vi "cal_trans.vi"(0 "Reference":T1, 3 "Input":T2) -> ()   [LabVIEW 2024]
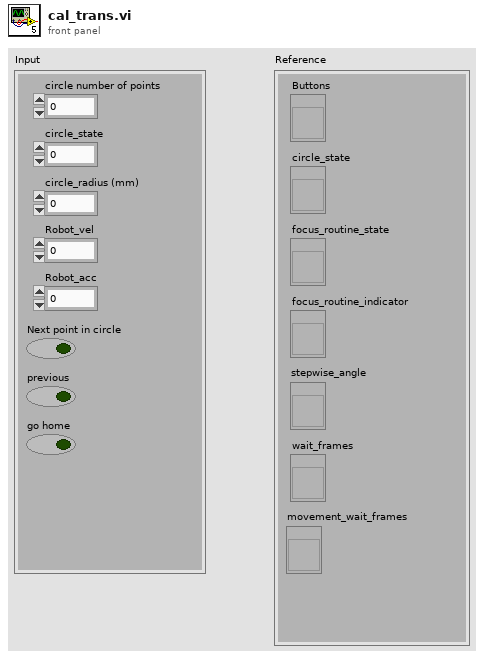
[diagram p1: front panel]
types:
  T1 = cluster{"Buttons":refnum<vi>, "circle_state":refnum<vi>, "focus_routine_state":refnum<vi>, "focus_routine_indicator":refnum<vi>, "stepwise_angle":refnum<vi>, "wait_frames":refnum<vi>, "movement_wait_frames":refnum<vi>}
  T2 = cluster{"circle number of points":i8, "circle_state":i8, "circle_radius (mm)":dbl, "Robot_vel":dbl, "Robot_acc":dbl, "Next point in circle":bool, "previous":bool, "go home":bool}
  T3 = cluster{"Focus routine":bool, "Freedrive mode":bool, "Next point in circle":bool, "previous":bool, "go home":bool}
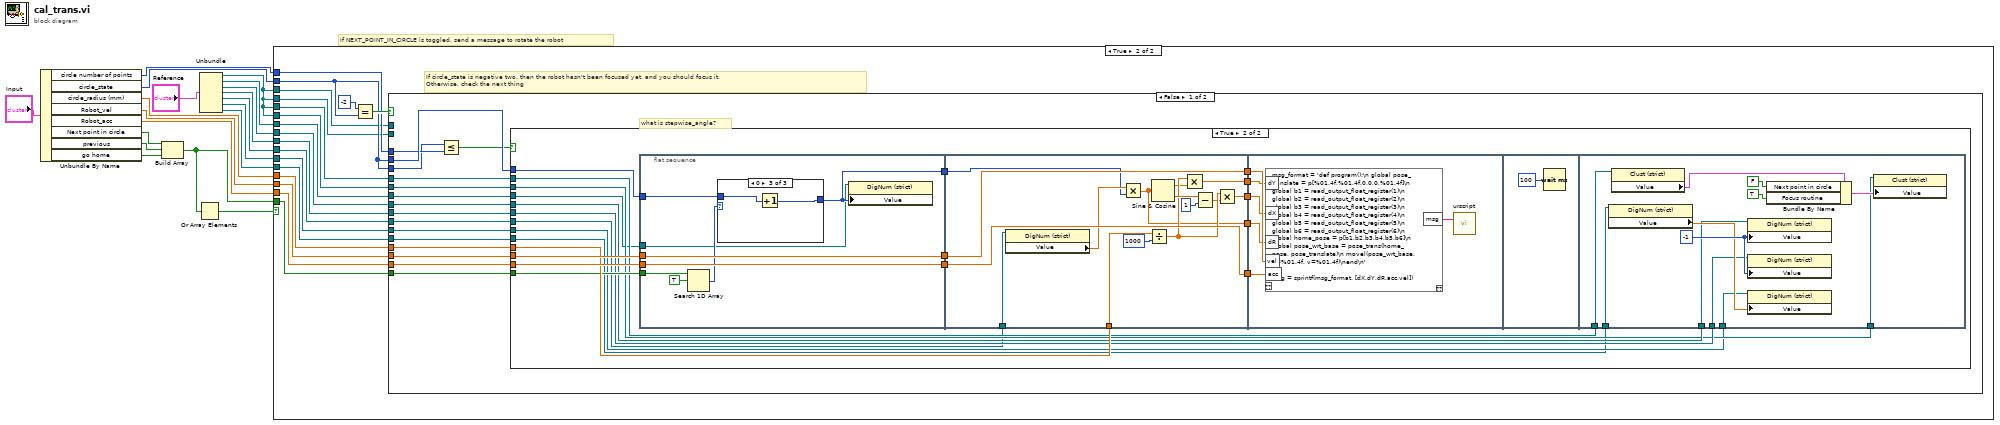
[diagram p0: block diagram]
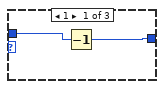
[diagram p4: hidden frame]
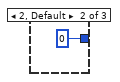
[diagram p5: hidden frame]
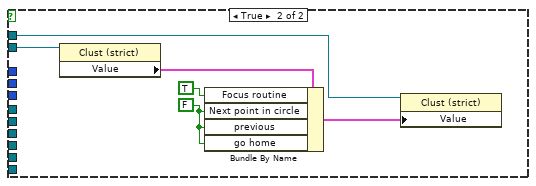
[diagram p6: hidden frame]
diagram:
  # "If NEXT_POINT_IN_CIRCLE is toggled, send a message to rotate the robot"
  n1 = Unbundle By Name("Input") -> ("circle number of points"=w16:i8, "circle_state"=w15:i8, "circle_radius (mm)"=w14:dbl, "Robot_vel"=w13:dbl, "Robot_acc"=w12:dbl, "Next point in circle"=w11:bool, "previous"=w9:bool, "go home"=w10:bool)
  n2 = Build Array(w11, w9, w10) -> (w19:bool[])
  n3 = Or Array Elements(Boolean array=w19) -> (logical OR=w18:bool)
  n4 = Unbundle("Reference") -> ("Buttons"=w7:refnum<vi>, "circle_state"=w6:refnum<vi>, "focus_routine_state"=w5:refnum<vi>, "focus_routine_indicator"=w4:refnum<vi>, "stepwise_angle"=w3:refnum<vi>, "wait_frames"=w2:refnum<vi>, "movement_wait_frames"=w1:refnum<vi>)
  n5 = case shown="True" w18 {
    tunnel: w15 -> [_ w32]
    tunnel: w16 -> [_ w35]
    tunnel: w13 -> [_ w34]
    tunnel: w12 -> [_ w33]
    tunnel: w14 -> [_ w31]
    tunnel: w19 -> [_ w30]
    tunnel: w5 -> [_ w29]
    tunnel: w4 -> [_ w28]
    tunnel: w7 -> [_ w27]
    tunnel: w2 -> [_ w26]
    tunnel: w1 -> [_ w25]
    tunnel: w7 -> [_ w24]
    tunnel: w3 -> [_ w23]
    tunnel: w6 -> [_ w22]
    tunnel: w7 -> [_ w21]
    tunnel: w7 -> [_ w20]
    frame False {
    }
    frame True {
      # "If circle_state is negative two, then the robot hasn't been focused yet, and you should focus it.\nOtherwise, check the next thing"
      n6 = Equal?(x=-2, y=w32) -> (x = y?=w36:bool)
      n7 = case shown="False" w36 {
        tunnel: w35 -> [w49 _]
        tunnel: w32 -> [w48 _]
        tunnel: w34 -> [w53 _]
        tunnel: w33 -> [w52 _]
        tunnel: w32 -> [w51 _]
        tunnel: w31 -> [w50 _]
        tunnel: w30 -> [w46 _]
        tunnel: w29 -> [w45 _]
        tunnel: w28 -> [w44 _]
        tunnel: w27 -> [w43 _]
        tunnel: w26 -> [w42 _]
        tunnel: w25 -> [w41 _]
        tunnel: w24 -> [w40 _]
        tunnel: w23 -> [w39 _]
        tunnel: w22 -> [w38 _]
        tunnel: w21 -> [_ w123]
        tunnel: w20 -> [_ w122]
        frame False {
          # "what is stepwise_angle?"
          n8 = Less Or Equal?(x=w48, y=w49) -> (x <= y?=w47:bool)
          n9 = case shown="True" w47 {
            tunnel: w53 -> [_ w74]
            tunnel: w52 -> [_ w73]
            tunnel: w51 -> [_ w64]
            tunnel: w50 -> [_ w65]
            tunnel: w46 -> [_ w62]
            tunnel: w45 -> [_ w61]
            tunnel: w44 -> [_ w60]
            tunnel: w43 -> [_ w59]
            tunnel: w42 -> [_ w58]
            tunnel: w41 -> [_ w57]
            tunnel: w40 -> [_ w56]
            tunnel: w39 -> [_ w55]
            tunnel: w38 -> [_ w54]
            frame False {
            }
            frame True {
              n10 = flat-sequence {
                tunnel: w64 -> [w80]
                tunnel: w73 -> [w81]
                tunnel: w74 -> [w82]
                tunnel: [w82] -> w67
                tunnel: [w81] -> w66
                tunnel: [w76] -> w63
                tunnel: w62 -> [w79]
                tunnel: w54 -> [w75]
                tunnel: [w102] -> w72
                tunnel: [w101] -> w71
                tunnel: [w90] -> w70
                tunnel: [w91] -> w69
                tunnel: [w92] -> w68
                tunnel: w67 -> [w102]
                tunnel: w66 -> [w101]
                tunnel: w65 -> [w94]
                tunnel: w63 -> [w89]
                tunnel: w55 -> [w88]
                tunnel: w72 -> [w108]
                tunnel: w71 -> [w107]
                tunnel: w70 -> [w106]
                tunnel: w69 -> [w105]
                tunnel: w68 -> [w104]
                tunnel: w61 -> [w115]
                tunnel: w60 -> [w114]
                tunnel: w59 -> [w113]
                tunnel: w58 -> [w112]
                tunnel: w57 -> [w111]
                tunnel: w56 -> [w110]
                frame #0 {
                  n11 = Search 1D Array(1D array=w79, element=TRUE) -> (index of element=w77:i32)  [unwired: 1 in]
                  n12 = case shown="0" w77 {
                    tunnel: w80 -> [w84 _ w87]
                    tunnel: [w83 0 w86] -> w76
                    frame 1 {
                      n13 = Decrement(x=w84) -> (x-1=w83:i8)
                    }
                    frame 2, Default {
                    }
                    frame 0 {
                      n14 = Increment(x=w87) -> (x+1=w86:i8)
                    }
                  }
                  n15 = property class="DigNum (strict)"(reference=w75, "Value"=w76) -> ()  [unwired: 1 in, 2 out]
                }
                frame #1 {
                  n16 = property class="DigNum (strict)"(reference=w88) -> ("Value"=w96:dbl)  [unwired: 1 in, 2 out]
                  n17 = Multiply(x=w96, y=w89) -> (x*y=w90:dbl)
                  n18 = Divide(x=w94, y=1000) -> (x/y=w99:dbl)
                  n19 = Sine & Cosine(0:w90) -> (1:w97:dbl, 2:w100:dbl)
                  n20 = Multiply(x=w99, y=w97) -> (x*y=w91:dbl)
                  n21 = Subtract(x=w100, y=1) -> (x-y=w98:dbl)
                  n22 = Multiply(x=w99, y=w98) -> (x*y=w92:dbl)
                }
                frame #2 {
                  n23 = script code="msg_format = 'def program():\\n global pose_translate = p[%01.4f,%01.4f,0,0,0,%01.4f]\\n global b1 = read_output_float_register(1)\\n global b2 = read_output_float_register(2)\\n global b3 = read_output_float_register(3)\\n global b4 = read_output_float_register(4)\\n global b5 = read_output_float_register(5)\\n global b6 = read_output_float_register(6)\\n global home_pose = p[b1,b2,b3,b4,b5,b6]\\n global pose_wrt_base = pose_trans(home_pose, pose_translate)\\n movel(pose_wrt_base, a=%01.4f, v=%01.4f)\\nend\\n'\n\nmsg = sprintf(msg_format, [dX,dY,dR,acc,vel])"("dX"=w104, "dY"=w105, "dR"=w106, "vel"=w108, "acc"=w107) -> ("msg"=w103:string)  [unwired: 1 in, 1 out]
                  n24 = call "urscript.vi"("String"=w103) -> ()  [unwired: 11 in]
                }
                frame #3 {
                  n25 = Wait (ms)(milliseconds to wait=100) -> ()  [unwired: 1 out]
                }
                frame #4 {
                  w121 = -1
                  n26 = property class="DigNum (strict)"(reference=w111) -> ("Value"=w120:dbl)  [unwired: 1 in, 2 out]
                  n27 = property class="Clust (strict)"(reference=w110) -> ("Value"=w118:T3)  [unwired: 1 in, 2 out]
                  n28 = property class="DigNum (strict)"(reference=w115, "Value"=w121) -> ()  [unwired: 1 in, 2 out]
                  n29 = property class="DigNum (strict)"(reference=w114, "Value"=w121) -> ()  [unwired: 1 in, 2 out]
                  n30 = property class="DigNum (strict)"(reference=w112, "Value"=w120) -> ()  [unwired: 1 in, 2 out]
                  n31 = Bundle By Name(cluster=w118, "Next point in circle"=FALSE, "Focus routine"=TRUE) -> (w119:T3)
                  n32 = property class="Clust (strict)"(reference=w113, "Value"=w119) -> ()  [unwired: 1 in, 2 out]
                }
              }
            }
          }
        }
        frame True {
          w124 = FALSE
          n33 = property class="Clust (strict)"(reference=w122) -> ("Value"=w125:T3)  [unwired: 1 in, 2 out]
          n34 = Bundle By Name(cluster=w125, "Focus routine"=TRUE, "Next point in circle"=w124, "previous"=w124, "go home"=w124) -> (w126:T3)
          n35 = property class="Clust (strict)"(reference=w123, "Value"=w126) -> ()  [unwired: 1 in, 2 out]
        }
      }
    }
  }
